vi "MUX_4to1.vi"(4 "Select":u8, 8 "Input 3":fxp<+/-,8,8>, 9 "Input 2":fxp<+/-,8,8>, 10 "Input 1":fxp<+/-,8,8>, 11 "Input 0":fxp<+/-,8,8>) -> (3 "Output":fxp<+/-,8,8>)   [LabVIEW 2015]
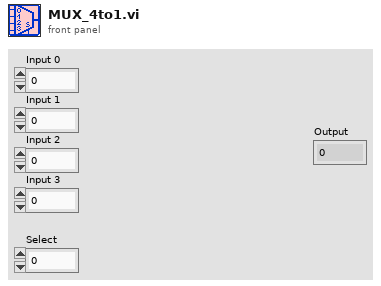
[diagram p1: front panel]
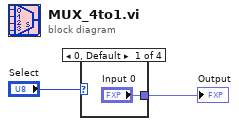
[diagram p0: block diagram]
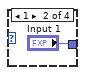
[diagram p2: hidden frame]
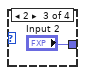
[diagram p3: hidden frame]
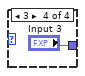
[diagram p4: hidden frame]
diagram:
  n1 = case shown="0, Default" "Select" {
    tunnel: ["Input 0" "Input 1" "Input 2" "Input 3"] -> w1
    frame 0, Default {
    }
    frame 1 {
    }
    frame 2 {
    }
    frame 3 {
    }
  }
  "Output" <- w1
